vi "Read Address.vi"(8 "error in":errorcluster, 11 "Element in":refnum<class "Element.lvclass">) -> (0 "error out":errorcluster, 2 "Address":i32[](array[numeric]), 3 "Element out":refnum<class "Element.lvclass">)   [LabVIEW 2014, in "Element.lvclass"]
uses:
  Element.lvclass
  Element.lvclass/Element.ctl
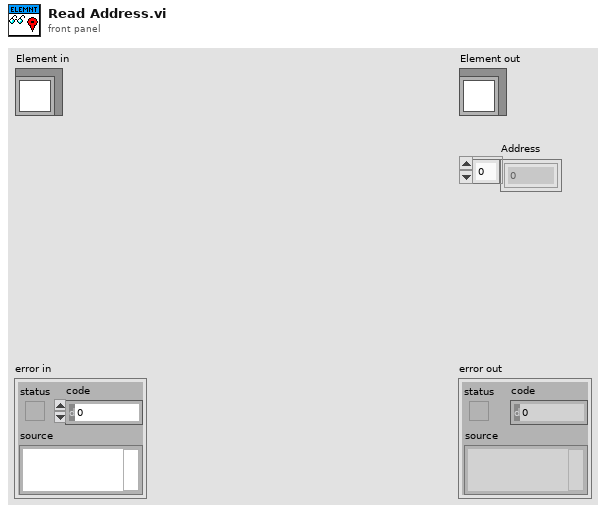
[diagram p1: front panel]
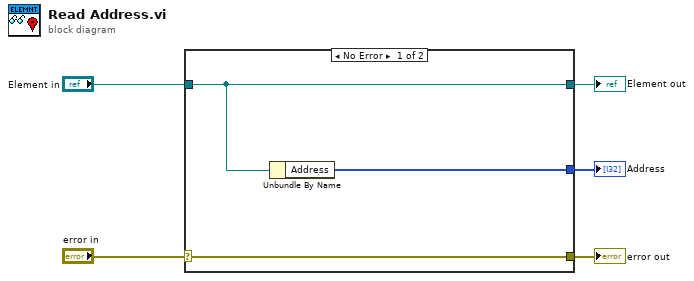
[diagram p0: block diagram]
diagram:
  n1 = case shown="No Error" "error in" {
    selector: "error in" -> [w8 w9]
    tunnel: [w8 w9] -> w4
    tunnel: [w7 w10] -> w2
    tunnel: "Element in" -> [w7 w10]
    tunnel: [w6 _] -> w1
    frame No Error {
      n2 = Unbundle By Name(w7) -> ("Address"=w6:i32[])
    }
    frame Error {
    }
  }
  "error out" <- w4
  "Element out" <- w2
  "Address" <- w1
